vi "Read Key.vi"(2 "健对象":string[](array[string]), 3 "Read section":string caption="查询段") -> (0 "未知健":bool, 1 "健值":string[](array[string]))   [LabVIEW 2014]
uses:
  <vilib>/Utility/config.llb/Read Key (String).vi
  <vilib>/Utility/config.llb/NI_LVConfig.lvlib
panel:
  out "error out 2":errorcluster caption="错误输出"
  out "error out":errorcluster caption="错误输出"
  out "查询结果":bool[](array[boolean])
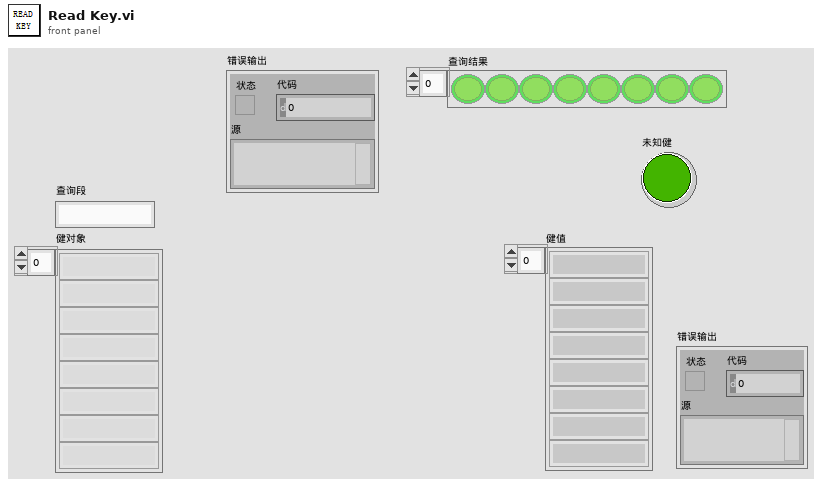
[diagram p1: front panel]
types:
  T1 = typedef "NI_LVConfig.lvlib/Config Data RefNum.ctl" = refnum<k1>
  T2 = cluster{"[0]":bool, "[1]":bool, "[2]":bool, "[3]":bool, "[4]":bool, "[5]":bool, "[6]":bool, "[7]":bool, "[8]":bool}
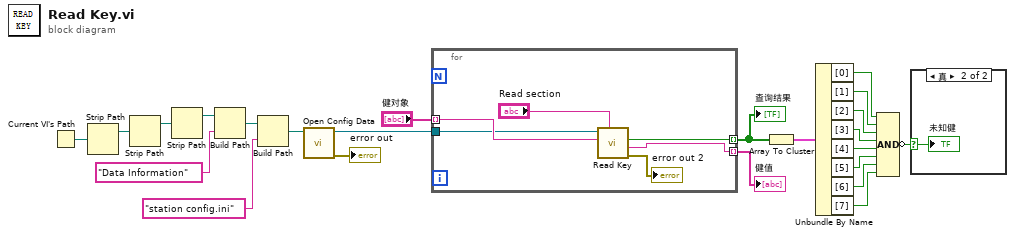
[diagram p0: block diagram]
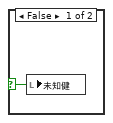
[diagram p2: hidden frame]
diagram:
  n1 = Current VI's Path() -> (path=w17:path)
  n2 = Strip Path(path=w17) -> (stripped path=w18:path)  [unwired: 1 out]
  n3 = Strip Path(path=w18) -> (stripped path=w22:path)  [unwired: 1 out]
  n4 = Strip Path(path=w22) -> (stripped path=w23:path)  [unwired: 1 out]
  n5 = Build Path(base path=w23, name or relative path="Data Information" ("名称或相对路径")) -> (appended path=w20:path)
  n6 = Build Path(base path=w20, name or relative path="station config.ini" ("名称或相对路径")) -> (appended path=w15:path)
  n7 = call <vilib>:"Open Config Data.vi"("configuration file path"=w15) -> ("error out"=→"error out":errorcluster, "refnum"=w14:T1)  [unwired: 8 in, 1 out]
  n8 = for {
    tunnel: "健对象" -> [w29] mode=indexing
    tunnel: w14 -> [w28]
    tunnel: [w24] -> w11 mode=indexing
    tunnel: [w27] -> w13 mode=indexing
    n9 = call-poly <vilib>:"Read Key.vi"("section"="Read section", "key"=w29, "refnum"=w28) -> ("error out"=→"error out 2":errorcluster, "value"=w27:string, "found?"=w24:bool)  [unwired: 5 in, 1 out]
  }
  "查询结果" <- w11
  "健值" <- w13
  n10 = Array To Cluster(array=w11) -> (cluster=w10:T2)
  n11 = Unbundle By Name(w10) -> ("[0]"=w9:bool, "[1]"=w8:bool, "[2]"=w7:bool, "[3]"=w6:bool, "[4]"=w5:bool, "[5]"=w4:bool, "[6]"=w3:bool, "[7]"=w2:bool)
  n12 = Compound Arithmetic op=AND(w9, w8, w7, w6, w5, w4, w3, w2) -> (invert w1:bool)
  n13 = case shown="真" w1 {
    selector: w1 -> [w30 w31]
    frame False {
      n14 = local write "未知健"(w30) -> ()
    }
    frame True {
      "未知健" <- w31
    }
  }
